vi "Plugin -Mid Offset.vi"(11 "Message Queues in":T2) -> ()   [LabVIEW 2019]
uses:
  support/Copy of Message Queue/All Message Queues.ctl
  support/Copy of Message Queue/Message Cluster.ctl
  controls/WhieBackgroundHistogram.ctl
  support/Copy of Message Queue/Copy of Message Queue.lvlib
panel:
  out "Time vs. Offset/Cor Offset":dbl(graph)
  out "Histogram Graph":T1
  out "T12":dbl(slide) scale=0.0..30.0
  out "T11":dbl(slide) scale=0.0..30.0
  out "T10":dbl(slide) scale=0.0..30.0
  out "T9":dbl(slide) scale=0.0..30.0
  out "T8":dbl(slide) scale=0.0..30.0
  out "T7":dbl(slide) scale=0.0..30.0
  out "T6":dbl(slide) scale=0.0..30.0
  out "T5":dbl(slide) scale=0.0..30.0
  out "T4":dbl(slide) scale=0.0..30.0
  out "T3":dbl(slide) scale=0.0..30.0
  out "T2":dbl(slide) scale=0.0..30.0
  out "T1":dbl(slide) scale=0.0..30.0
  out "Ring Time":waveform(dbl)[](graph)
  out "Aquatrak RS232 Output":string
  in  "error in":errorcluster
  out "error out":errorcluster
  # "Calulating Short Offset"
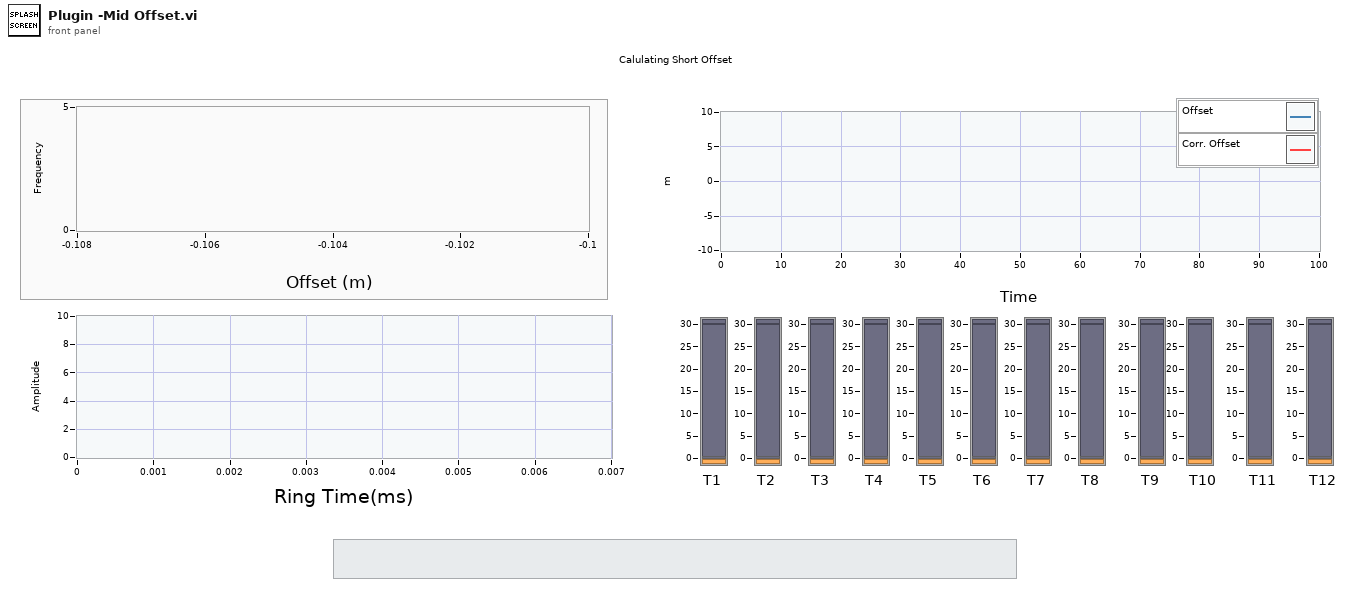
[diagram p1: front panel]
types:
  T1 = typedef "WhieBackgroundHistogram.ctl" = cluster{"X Values":dbl[], "Histogram: h(x)":i32[]}
  T2 = typedef "Copy of Message Queue.lvlib/All Message Queues.ctl" = cluster{"UI":refnum<queue>, "Acquisition":refnum<queue>, "Logging":refnum<queue>, "Analyze":refnum<queue>}
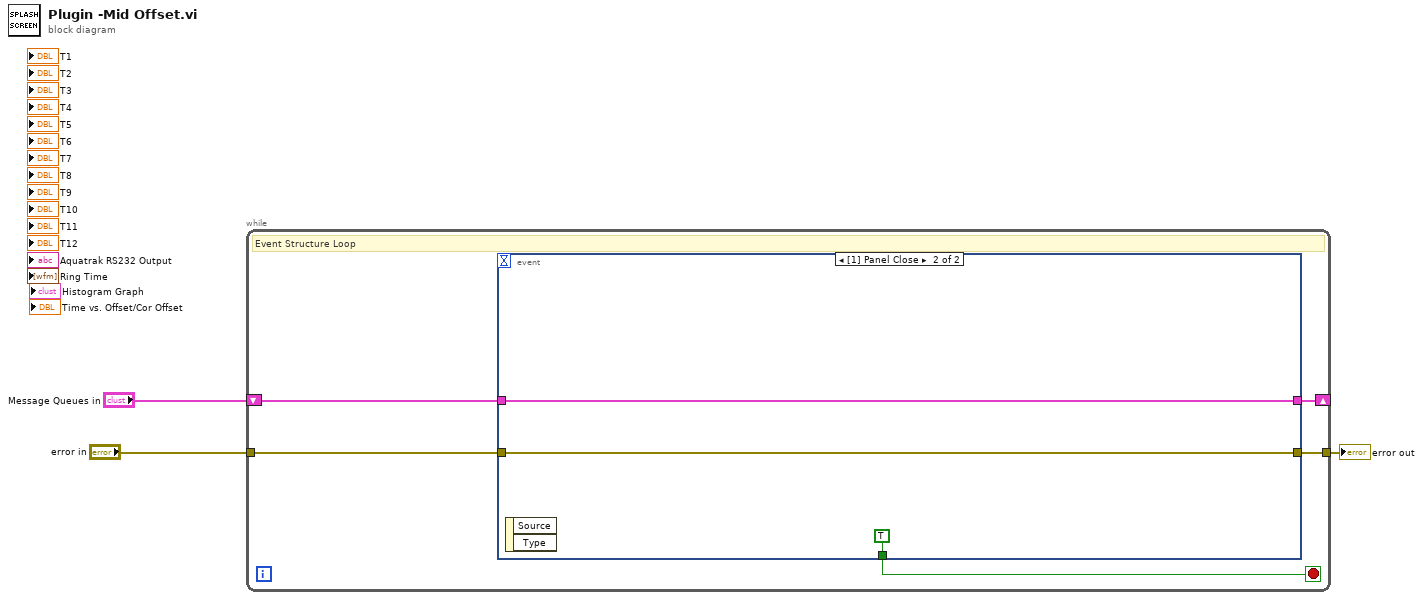
[diagram p0: block diagram]
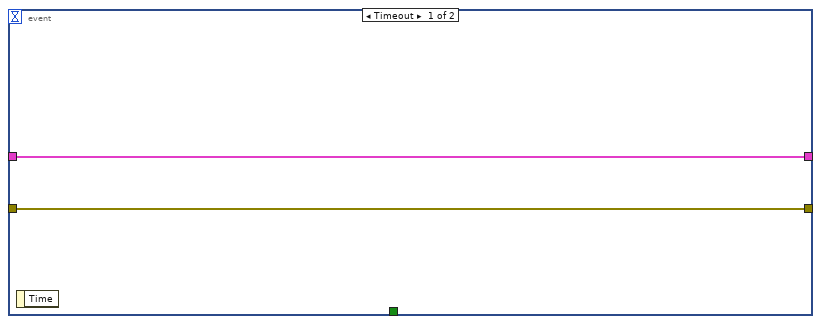
[diagram p2: hidden frame]
diagram:
  n1 = while {
    shift-right: [w7] -> _
    shift-left: "Message Queues in" -> [w6]
    tunnel: [w5] -> w2
    tunnel: "error in" -> [w4]
    stop <- w8 stop-if-true
    # "Event Structure Loop"
    n2 = event shown="[1] Panel Close" {
      selector: _ -> [_ _]
      dyn-events: _ -> [_ _]
      timeout: _ -> [_ _]
      tunnel: [_ TRUE ("NewVal")] -> w8
      tunnel: w6 -> [w10 w13]
      tunnel: [w10 w13] -> w7
      tunnel: [w9 w11] -> w5
      tunnel: w4 -> [w9 w11]
      event Timeout {
        n3 = event-data() -> ()  [unwired: 1 in, 1 out]
      }
      event Panel Close {
        n4 = event-data() -> ()  [unwired: 1 in, 2 out]
      }
    }
  }
  "error out" <- w2
